vi "ToString.vi"(8 "error in (no error)":errorcluster, 11 "U32 D Element in":refnum<class "U8 D Element.lvclass">) -> (0 "error out":errorcluster, 2 "String":string, 3 "U32 D Element out":refnum<class "U8 D Element.lvclass">)   [LabVIEW 2018, in "D Datagrid Library.lvlib" / "U8 D Element.lvclass"]
uses:
  U8 D Element.lvclass
  U8 D Element.lvclass/U8 D Element.ctl
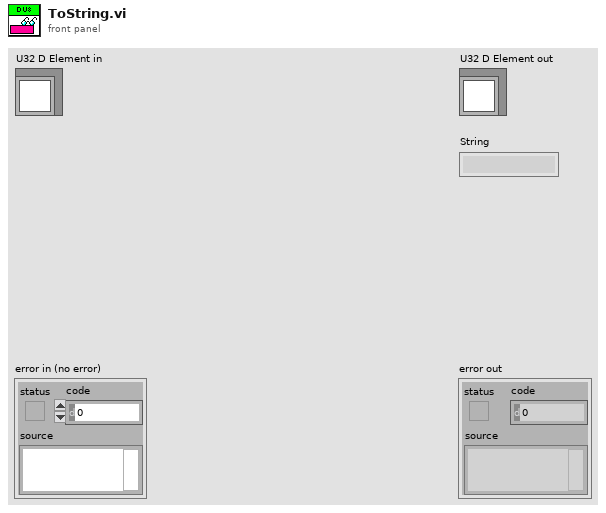
[diagram p1: front panel]
types:
  T1 = typedef "D Datagrid Library.lvlib/U8 D Element.lvclass/Display mode.ctl" = enum16{"Standard", "Hex"}
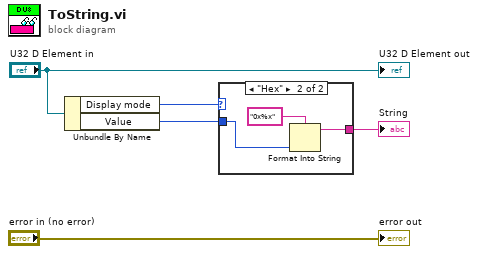
[diagram p0: block diagram]
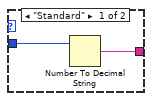
[diagram p2: hidden frame]
diagram:
  n1 = Unbundle By Name("U32 D Element in") -> ("Display mode"=w1:T1, "Value"=w3:u8)
  n2 = case shown="\"Hex\"" w1 {
    tunnel: w3 -> [w7 w10]
    tunnel: [w6 w9] -> w2
    frame "Standard" {
      n3 = Number To Decimal String(number=w7) -> (decimal integer string=w6:string)  [unwired: 1 in]
    }
    frame "Hex" {
      n4 = Format Into String(format string="0x%x", w10) -> (resulting string=w9:string)  [unwired: 2 in, 1 out]
    }
  }
  "String" <- w2
  "error out" <- "error in (no error)"
  "U32 D Element out" <- "U32 D Element in"
